vi "hse-application_SelectProjectFolder.vi"(8 "error in":errorcluster, 10 "Start path":path) -> (0 "error out":errorcluster, 2 "PROJECT Folder":path, 3 "PROJECT Name":string)   [LabVIEW 2020, in "hse-application.lvclass"]
doc: "Opens a file dialog to select the folder in which the project file and the startup.vi are located.\n\n____\nHAMPEL SOFTWARE ENGINEERING v3.8.0 (2023-12-18 14:41)"
uses:
  hse-application.lvclass
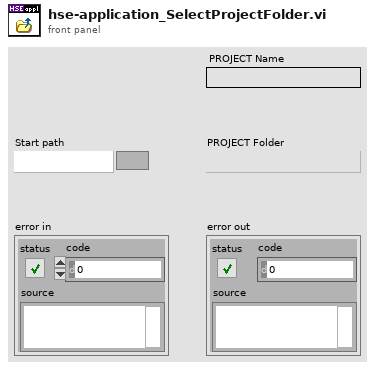
[diagram p1: front panel]
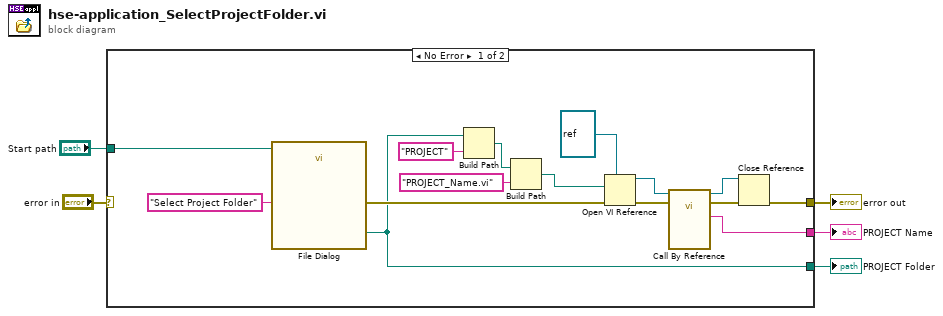
[diagram p0: block diagram]
diagram:
  n1 = case shown="No Error" "error in" {
    selector: "error in" -> [_ w21]
    tunnel: [w16 _] -> w3
    tunnel: "Start path" -> [w10 _]
    tunnel: [w17 w21] -> w5
    tunnel: [w8 _] -> w1
    frame No Error {
      n2 = call "File Dialog"("start path"=w10, "prompt"="Select Project Folder") -> ("selected path"=w8:path, "error out"=w20:errorcluster)  [unwired: 10 in, 2 out]
      n3 = Build Path(base path=w8, name or relative path="PROJECT") -> (appended path=w12:path)
      n4 = Build Path(base path=w12, name or relative path="PROJECT_Name.vi") -> (appended path=w6:path)
      n5 = Open VI Reference(type specifier VI Refnum (for type only)=refnum<vi> refnum, vi path=w6, error in (no error)=w20) -> (vi reference=w14:refnum<vi>, error out=w19:errorcluster)  [unwired: 3 in]
      n6 = call-by-ref "Call By Reference"(reference=w14, error in=w19) -> (reference out=w9:refnum<vi>, error out=w18:errorcluster, "PROJECT Name"=w16:string)  [unwired: 11 in]
      n7 = Close Reference(reference=w9, error in (no error)=w18) -> (error out=w17:errorcluster)
    }
    frame Error {
    }
  }
  "PROJECT Folder" <- w1
  "PROJECT Name" <- w3
  "error out" <- w5
